vi "update_RF_generators.vi"(8 "error in":errorcluster, 11 "GPIB (in)":refnum<class "GPIB.lvclass">) -> (0 "error out":errorcluster, 3 "GPIB":refnum<class "GPIB.lvclass">)   [LabVIEW 2013, in "GPIB.lvclass"]
uses:
  GPIB.lvclass
  GPIB.lvclass/GPIB.ctl
  HP83623A_RF_Generator/HP83623A_RF_Generator.lvclass
  HP83712B_RF_Generator/HP83712B_RF_Generator.lvclass
  HP8662A_RF_Generator/HP8662A_RF_Generator.lvclass
  Globals.vi
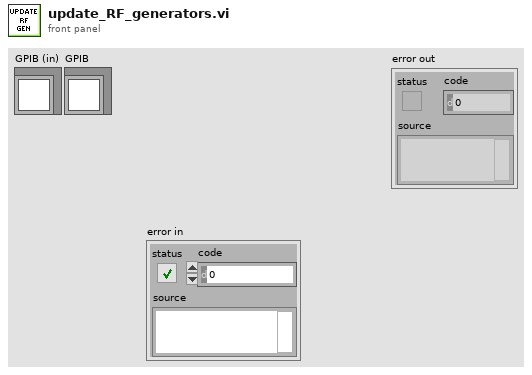
[diagram p1: front panel]
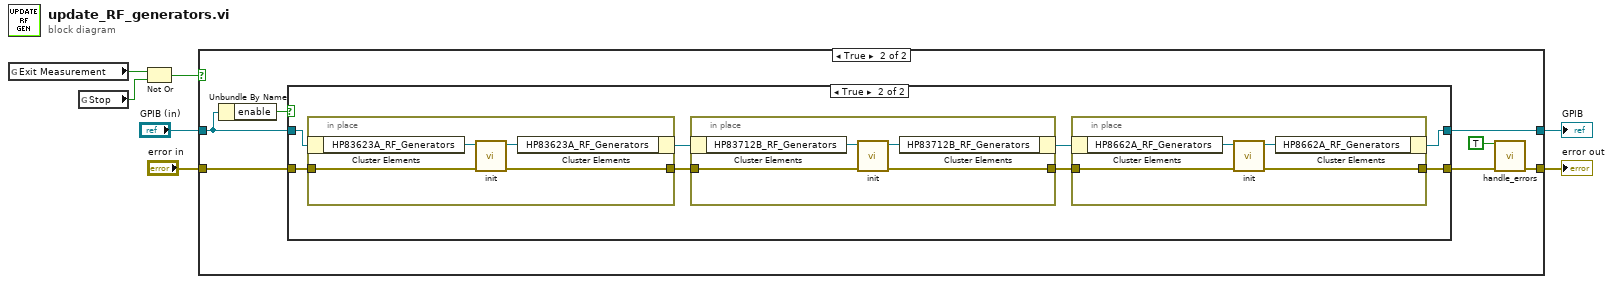
[diagram p0: block diagram]
diagram:
  n1 = global read "Globals.vi" "Exit Measurement"() -> (w3:bool)
  n2 = global read "Globals.vi" "Stop"() -> (w2:bool)
  n3 = Not Or(1:w2, 2:w3) -> (0:w1:bool)
  n4 = case shown="True" w1 {
    tunnel: "error in" -> [w8 w16]
    tunnel: "GPIB (in)" -> [w9 w13]
    tunnel: [w9 w15] -> w5
    tunnel: [w8 w10] -> w4
    frame False {
    }
    frame True {
      n5 = Unbundle By Name(w13) -> ("enable"=w12:bool)
      n6 = case shown="True" w12 {
        tunnel: w16 -> [w17 w26]
        tunnel: w13 -> [w18 w25]
        tunnel: [w18 w21] -> w15
        tunnel: [w17 w19] -> w11
        frame False {
        }
        frame True {
          n7 = in-place {
            in-place-border: w26 -> [w38]
            in-place-border: [w35] -> w23
            n8 = in-place-cluster #1(w25) -> ("HP83623A_RF_Generators"=w37:refnum<class "HP83623A_RF_Generator.lvclass">)
            n9 = call-dynamic "init.vi"("error in (no error)"=w38, "HP83623A_RF_Generator in"=w37) -> ("error out"=w35:errorcluster, "HP83623A_RF_Generator out"=w36:refnum<class "HP83623A_RF_Generator.lvclass">)  [unwired: 8 in]
            n10 = in-place-cluster #1("HP83623A_RF_Generators"=w36) -> (w24:refnum<class "GPIB.lvclass">)
          }
          n11 = in-place {
            in-place-border: w23 -> [w32]
            in-place-border: [w31] -> w20
            n12 = in-place-cluster #2(w24) -> ("HP83712B_RF_Generators"=w34:refnum<class "HP83712B_RF_Generator.lvclass">)
            n13 = call-dynamic "init.vi"("error in (no error)"=w32, "HP83712B_RF_Generator in"=w34) -> ("error out"=w31:errorcluster, "HP83712B_RF_Generator out"=w33:refnum<class "HP83712B_RF_Generator.lvclass">)  [unwired: 8 in]
            n14 = in-place-cluster #2("HP83712B_RF_Generators"=w33) -> (w22:refnum<class "GPIB.lvclass">)
          }
          n15 = in-place {
            in-place-border: w20 -> [w30]
            in-place-border: [w27] -> w19
            n16 = in-place-cluster #3(w22) -> ("HP8662A_RF_Generators"=w29:refnum<class "HP8662A_RF_Generator.lvclass">)
            n17 = call-dynamic "init.vi"("error in (no error)"=w30, "HP8662A_RF_Generator in"=w29) -> ("error out"=w27:errorcluster, "HP8662A_RF_Generator out"=w28:refnum<class "HP8662A_RF_Generator.lvclass">)  [unwired: 8 in]
            n18 = in-place-cluster #3("HP8662A_RF_Generators"=w28) -> (w21:refnum<class "GPIB.lvclass">)
          }
        }
      }
      n19 = call "handle_errors.vi"("Exit Operation"=TRUE ("Exit Measurement"), "error in (no error)"=w11) -> ("error out"=w10:errorcluster)  [unwired: 13 in]
    }
  }
  "error out" <- w4
  "GPIB" <- w5
